vi "PP.PNG.File.Encode.vi"(5 "Password":string, 7 "error in":errorcluster, 9 "File Path":path, 10 "PNG In":path) -> (0 "error out":errorcluster)   [LabVIEW 2020, in "PixPack.lvlib"]
uses:
  private/User.Encode.Format.ctl
  PixPack.lvlib
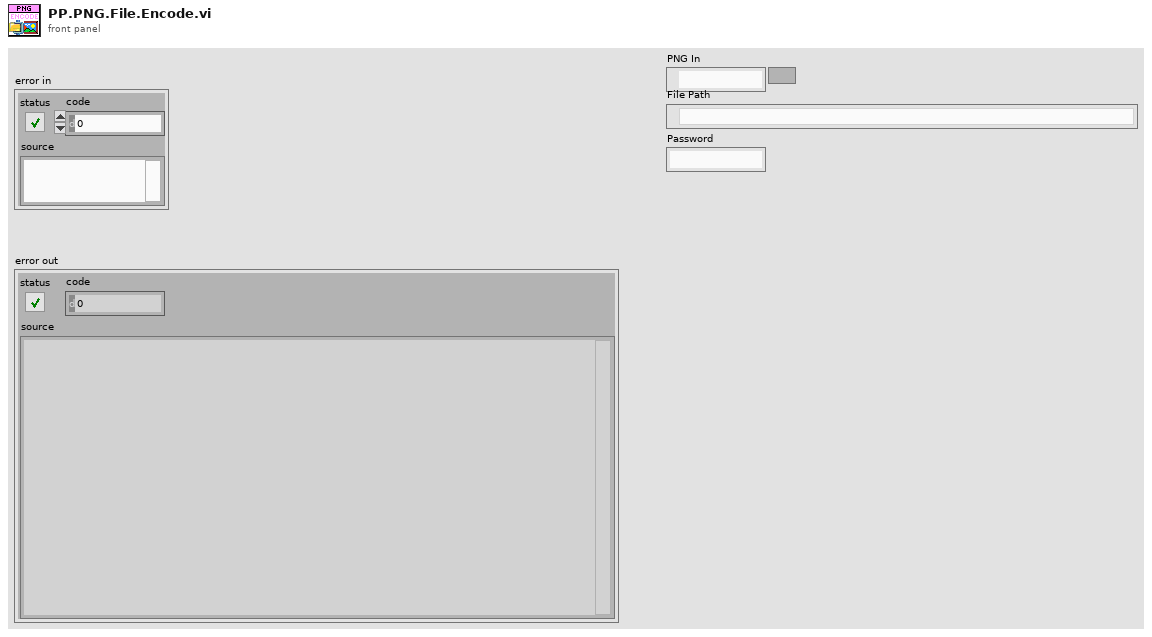
[diagram p1: front panel]
types:
  T1 = typedef "PixPack.lvlib/User.Encode.Format.ctl" = enum16{"XML Encode", "Normal Flatten", "External File"}
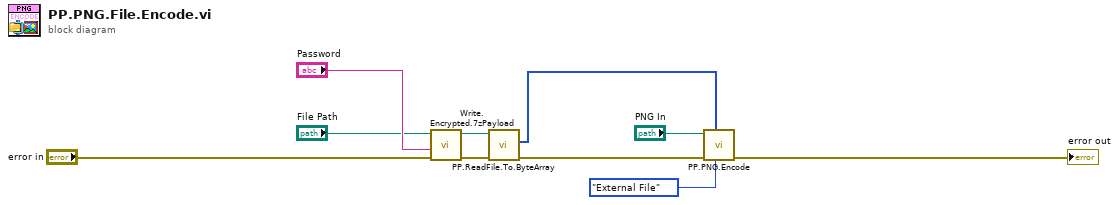
[diagram p0: block diagram]
diagram:
  n1 = call "Write.Encrypted.7zPayload.vi"("error in (no error)"="error in", "Password"="Password", "File Path"="File Path") -> ("error out"=w8:errorcluster, "7z Path Out"=w7:path)  [unwired: 7 in]
  n2 = call "PP.ReadFile.To.ByteArray.vi"("error in"=w8, "file path (use dialog)"=w7) -> ("error out"=w1:errorcluster, "data"=w10:u8[])  [unwired: 7 in, 1 out]
  n3 = call "PP.PNG.Encode.vi"("Encode Format"=User.Encode.Format."External File", "Data"=w10, "error in"=w1, "PNG In"="PNG In") -> ("error out"=→"error out":errorcluster)  [unwired: 7 in]
